vi "Read Car Wash Controller.vi"(8 "error in (no error)":errorcluster, 11 "Wash Display Console in":refnum<class "Wash Display Console.lvclass">) -> (0 "error out":errorcluster, 2 "Architecture.lvlib:Queue.lvclass":refnum<class "Queue.lvclass">, 3 "Wash Display Console out":refnum<class "Wash Display Console.lvclass">)   [LabVIEW 2016, in "Wash Display Console.lvlib" / "Wash Display Console.lvclass"]
uses:
  Wash Display Console.lvclass
  Queue/Queue.lvclass
  Wash Display Console.lvclass/Wash Display Console.ctl
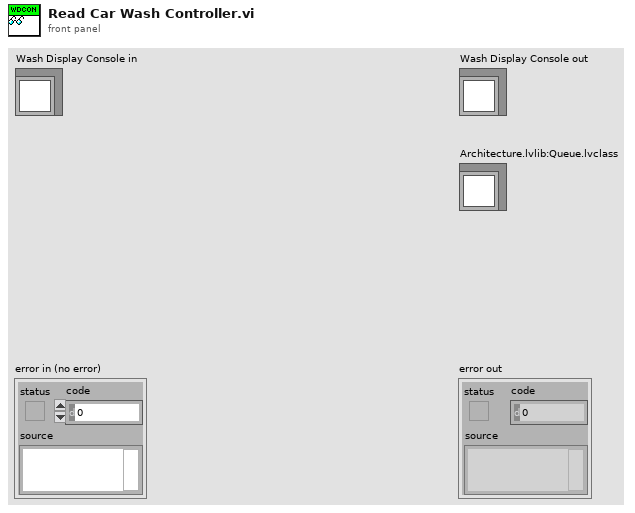
[diagram p1: front panel]
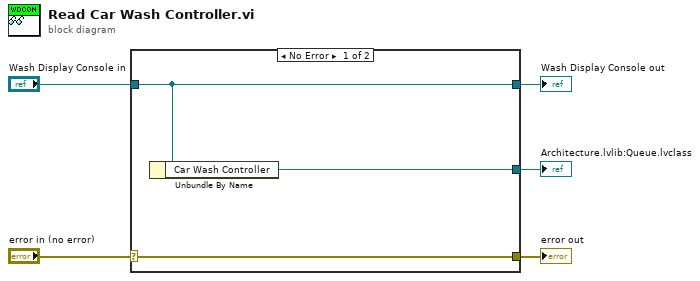
[diagram p0: block diagram]
diagram:
  n1 = case shown="No Error" "error in (no error)" {
    selector: "error in (no error)" -> [w8 w9]
    tunnel: [w8 w9] -> w4
    tunnel: [w7 w10] -> w2
    tunnel: "Wash Display Console in" -> [w7 w10]
    tunnel: [w6 _] -> w1
    frame No Error {
      n2 = Unbundle By Name(w7) -> ("Car Wash Controller"=w6:refnum<class "Queue.lvclass">)
    }
    frame Error {
    }
  }
  "error out" <- w4
  "Wash Display Console out" <- w2
  "Architecture.lvlib:Queue.lvclass" <- w1
